vi "Timeout Selector.vi"(6 "Remaining States":string, 7 "Timeout Expected":i32) -> (3 "Timeout":i32)   [LabVIEW 2017, in "Communicable State Machine.lvlib"]
doc: "#### Timeout Selector.vi\n\nUsed in templates with a user event structure.\n\n-- <b>Controls</b> --\n- <b>Timeout Expected</b>: Expected timeout setting\n- <b>Remaining States</b>: Outputs 0 if there are remaining states; otherwise, outputs the expected value\n\n-- <b>Indicators</b> --\n- <b>Timeout</b>: Timeout setting after arbitration"
uses:
  Communicable State Machine.lvlib
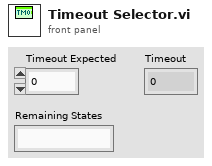
[diagram p1: front panel]
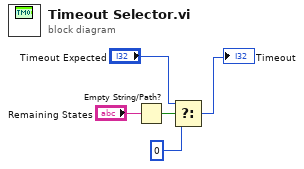
[diagram p0: block diagram]
diagram:
  n1 = Empty String/Path?(string/path="Remaining States") -> (empty?=w2:bool)
  n2 = Select(t="Timeout Expected", s=w2, f=0) -> (s? t:f=→"Timeout":i32)
